vi "LEP_RV_LaunchGlobals.vi"() -> ()   [LabVIEW 2011]
uses:
  LEP_RV_Config.ctl
panel:
  in  "Remember password":bool
  in  "Password":string
  in  "User name":string
  in  "Compiler server name":string
  in  "Connect to a network compile server":bool
  in  "Client installed":bool
  out "Active File Count":i32
  in  "embeddedSessionID":u32
  in  "Use Global":bool
  in  "vi reference":refnum<vi>
  in  "Root ID":string
  in  "Item ID":string
  in  "build ID":u32
  in  "target ID":u32
  in  "MaxElements":u32
  in  "UpdateClusters":u32
  in  "UpdateArrays":u32
  in  "Update":u32
  in  "DebugSerialBaud":u32
  in  "DebugSerialPort":string
  in  "BreakpointsConfig":cluster{"Clear on Start":bool}
  in  "File List":path[](array[path])
  in  "buildSpec ID":string
  in  "TopLevelVI":path
  in  "Build Path":path
  in  "Config":T1={"Enable debugging"=FALSE, "Debug Options"=0, "Use stack variables"=FALSE, "Generate serial only"=FALSE, "Generate guard code"=FALSE, "Generate Integer Only"=FALSE, "Generate C Function Calls"=TRUE, "ExpressionFolding"=TRUE, "Constant Allocation"=0, "Constant Deallocation"=0, "Build Specification ID"="", "Preprocessor symbols (define)"="", "Compiler Flags"="", "Linker Flags"="", "Mode"=1, "Optimization"=2, "Optimize for time"=FALSE, "Enable cross-module optimization"=FALSE, "Include paths"=[], "Optimize heap size"=TRUE, "Use MicroLib"=FALSE, "Debug Mode"=2, "Enable profile information"=FALSE, "Host name"="board", "Use DHCP"=TRUE, "IP address"="0.0.0.0", "Subnet mask"="", "Gateway"="0.0.0.0", "Primary DNS"="0.0.0.0", "Secondary DNS"="0.0.0.0", "MAC in target memory"=TRUE, "MAC address"="", "Console output"=1, "Target serial port"=1} {"Constant Deallocation" items=["Out of Scope", "VI End", "Application End"]; "Constant Allocation" items=["First Use", "Containing Loop", "VI Initialization", "Application Initialization"]; "Target serial port" items=["0", "1", "2", "3"]; "Console output" items=["Processor status window", "Serial port"]; "Optimization" items=["Level 0 (-O0)", "Level 1 (-O1)", "Level 2 (-O2)", "Level 3 (-O3)"]; "Mode" items=["ARM-Mode", "Thumb-Mode"]; "Debug Options" items=["Use ULINK Debugger", "Use Simulator"]; "Debug Mode" items=["Instrumented (serial port)", "Instrumented (TCP/IP)", "Non-instrumented (JTAG/USB)"]}
  in  "UV License OK":bool
  in  "UV Project File":path
  in  "Target Name":string
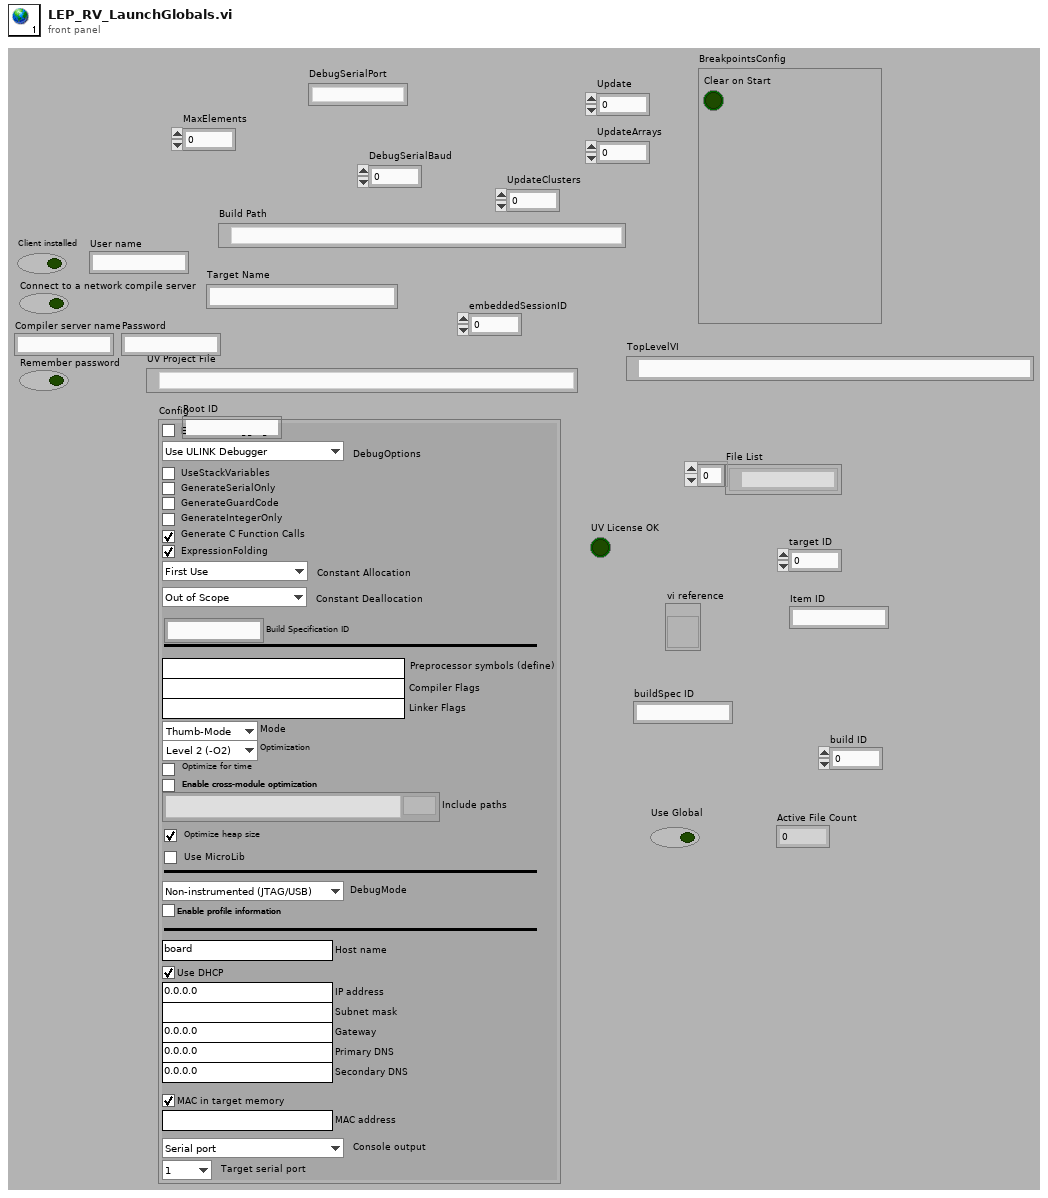
[diagram p1: front panel]
types:
  T1 = typedef "LEP_RV_Config.ctl" = cluster{"Enable debugging":bool, "Debug Options":u16, "Use stack variables":bool, "Generate serial only":bool, "Generate guard code":bool, "Generate Integer Only":bool, "Generate C Function Calls":bool, "ExpressionFolding":bool, "Constant Allocation":u16, "Constant Deallocation":u16, "Build Specification ID":string, "Preprocessor symbols (define)":string, "Compiler Flags":string, "Linker Flags":string, "Mode":u16, "Optimization":u16, "Optimize for time":bool, "Enable cross-module optimization":bool, "Include paths":path[], "Optimize heap size":bool, "Use MicroLib":bool, "Debug Mode":u16, "Enable profile information":bool, "Host name":string, "Use DHCP":bool, "IP address":string, "Subnet mask":string, "Gateway":string, "Primary DNS":string, "Secondary DNS":string, "MAC in target memory":bool, "MAC address":string, "Console output":u16, "Target serial port":u16}
diagram:
